vi "CSM - Replace Substitution Marks in Messages.vi"(5 "States with Replace Token":string, 7 "<param>":string, 9 "<target>":string, 12 "<1>":string, 13 "<2>":string) -> (6 "States":string)   [LabVIEW 2020, in "Communicable State Machine.lvlib"]
uses:
  Communicable State Machine.lvlib
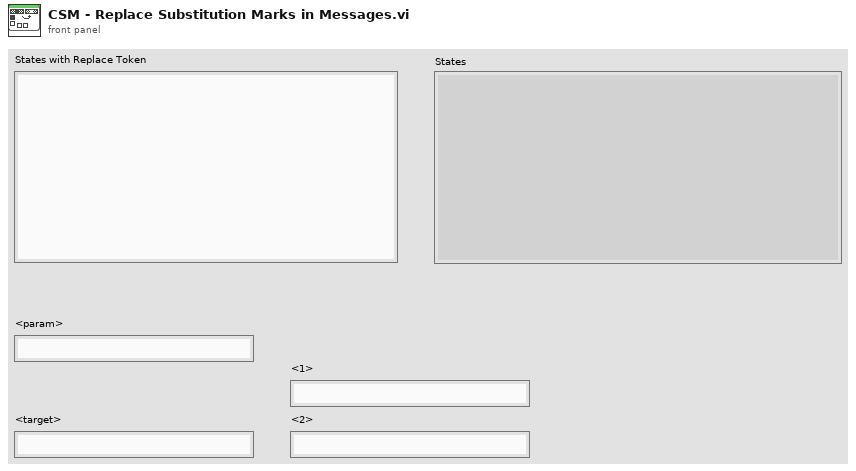
[diagram p1: front panel]
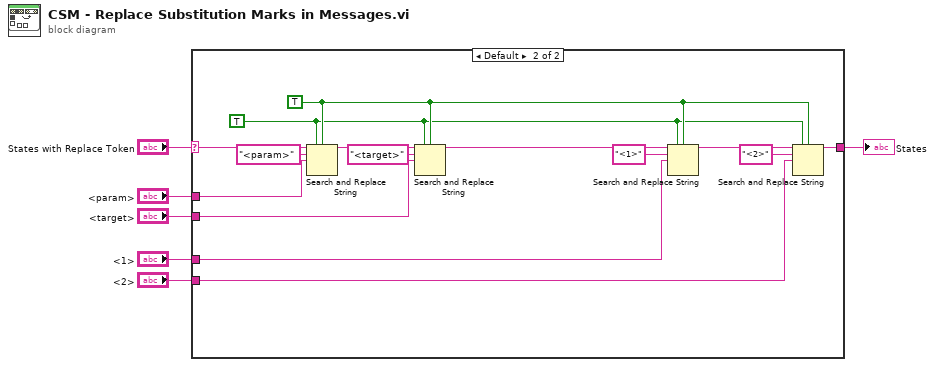
[diagram p0: block diagram]
diagram:
  n1 = case shown="Default" "States with Replace Token" {
    selector: "States with Replace Token" -> [w7 w22]
    tunnel: "<param>" -> [_ w21]
    tunnel: "<target>" -> [_ w20]
    tunnel: [w7 w12] -> w5
    tunnel: "<2>" -> [_ w9]
    tunnel: "<1>" -> [_ w8]
    frame "" {
    }
    frame Default {
      w11 = TRUE ("ignore case? (F)")
      w10 = TRUE ("replace all? (F)")
      n2 = Search and Replace String(replace all?=w10, case sensitive?=w11, input string=w22, search string="<param>", replace string=w21) -> (result string=w19:string)  [unwired: 3 in, 3 out]
      n3 = Search and Replace String(replace all?=w10, case sensitive?=w11, input string=w19, search string="<target>", replace string=w20) -> (result string=w18:string)  [unwired: 3 in, 3 out]
      n4 = Search and Replace String(replace all?=w10, case sensitive?=w11, input string=w18, search string="<1>", replace string=w8) -> (result string=w13:string)  [unwired: 3 in, 3 out]
      n5 = Search and Replace String(replace all?=w10, case sensitive?=w11, input string=w13, search string="<2>", replace string=w9) -> (result string=w12:string)  [unwired: 3 in, 3 out]
    }
  }
  "States" <- w5
